vi "set_undocked_status.vi"(8 "error in (no error)":errorcluster, 10 "has undocked window?":bool, 11 "DisplayDL090216 in":refnum<class "DisplayDL090216.lvclass">) -> (0 "error out":errorcluster, 3 "DisplayDL090216 out":refnum<class "DisplayDL090216.lvclass">)   [LabVIEW 2010, in "DisplayDL090216.lvclass"]
uses:
  DisplayDL090216.lvclass
  DisplayDL090216.lvclass/DisplayDL090216.ctl
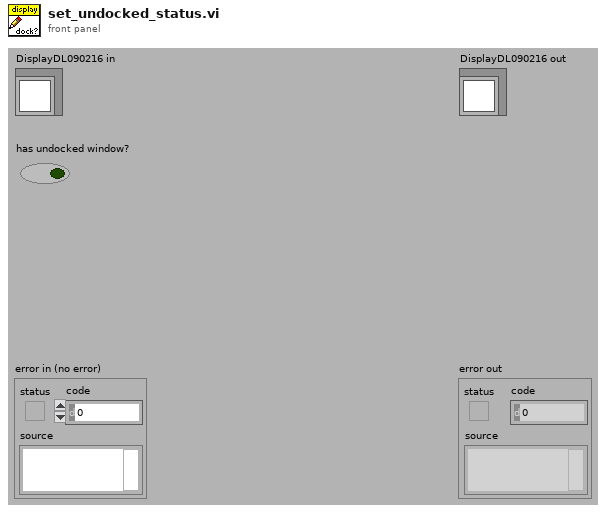
[diagram p1: front panel]
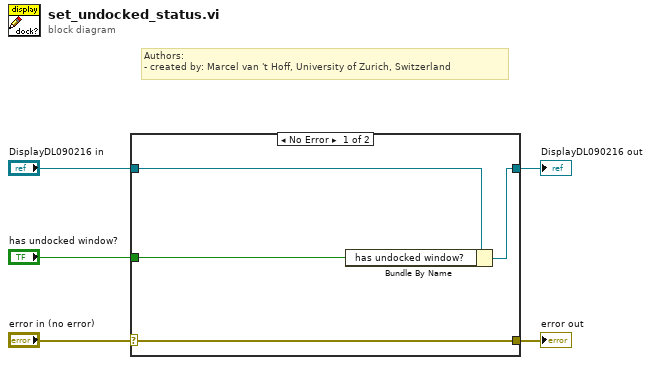
[diagram p0: block diagram]
diagram:
  # "Authors: \n- created by: Marcel van 't Hoff, University of Zurich, Switzerland"
  n1 = case shown="No Error" "error in (no error)" {
    selector: "error in (no error)" -> [w9 w10]
    tunnel: [w9 w10] -> w4
    tunnel: [w7 w11] -> w2
    tunnel: "DisplayDL090216 in" -> [w8 w11]
    tunnel: "has undocked window?" -> [w6 _]
    frame No Error {
      n2 = Bundle By Name(cluster=w8, "has undocked window?"=w6) -> (w7:refnum<class "DisplayDL090216.lvclass">)
    }
    frame Error {
    }
  }
  "error out" <- w4
  "DisplayDL090216 out" <- w2
